vi "Update Plugin Types.vi"(8 "error in (no error)":errorcluster, 10 "plugin_types":T1[](array[typedef]), 11 "Plugin Types ref in":refnum<vi>) -> (0 "error out":errorcluster, 3 "Plugin Types ref out":refnum<vi>)   [LabVIEW 2021, in "CIF_UI.lvclass"]
uses:
  CIF_UI.lvclass
  CIF_UI.lvclass/CIF_UI.ctl
  CIFPluginManager/CIFPluginManager/gRPC/CIF_Manager_client/RPC Messages/cif_manager_PluginVersion.ctl
  CIFPluginManager/CIFPluginManager/gRPC/CIF_Manager_client/CIF_Manager_client.lvlib
  CIFPluginManager/CIFPluginManager/gRPC/CIF_Manager_client/RPC Messages/cif_manager_PluginType.ctl
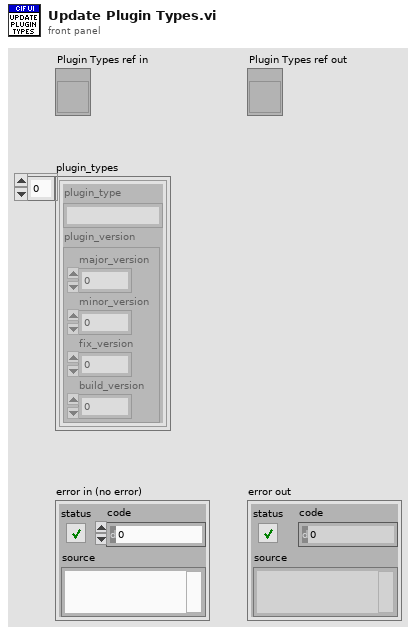
[diagram p1: front panel]
types:
  T1 = typedef "CIF_Manager_client.lvlib/cif_manager_PluginType.ctl" = cluster{"plugin_type":string, "plugin_version":T2}
  T2 = typedef "CIF_Manager_client.lvlib/cif_manager_PluginVersion.ctl" = cluster{"major_version":i32, "minor_version":i32, "fix_version":i32, "build_version":i32}
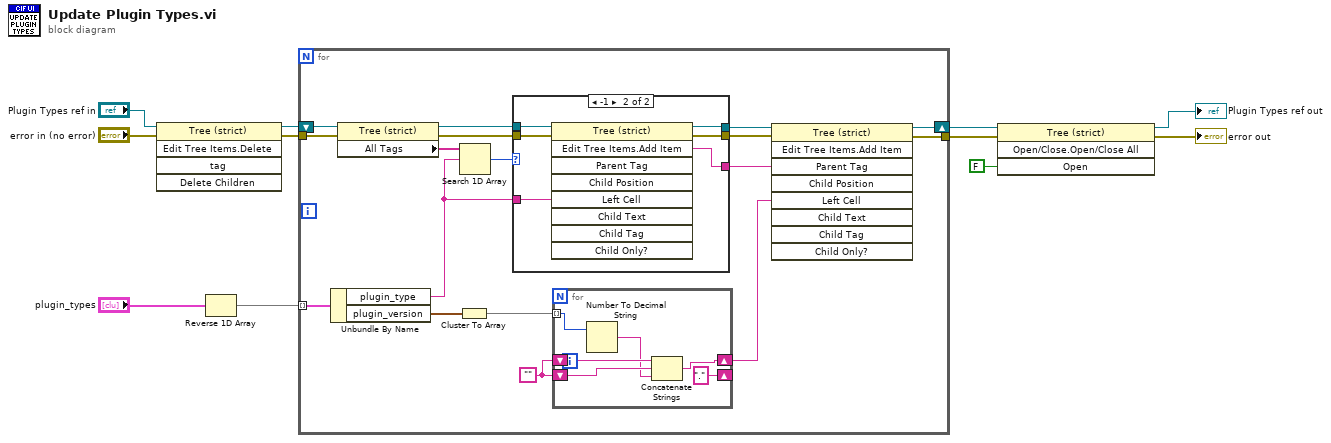
[diagram p0: block diagram]
diagram:
  n1 = invoke class="Tree (strict)" method="Edit Tree Items.Delete"(reference="Plugin Types ref in", error in="error in (no error)") -> (reference out=w10:refnum<vi>, error out=w11:errorcluster)  [unwired: 3 in, 3 out]
  n2 = Reverse 1D Array(array="plugin_types") -> (reversed array=w1:T1[])
  n3 = for {
    tunnel: w11 -> [w17]
    tunnel: [w27] -> w8
    tunnel: w1 -> [w25] mode=indexing
    shift-right: [w12] -> w9
    shift-left: w10 -> [w18]
    w22 = ""
    n4 = Unbundle By Name(w25) -> ("plugin_type"=w20:string, "plugin_version"=w24:T2)
    n5 = property class="Tree (strict)"(reference=w18, error in=w17) -> (reference out=w14:refnum<vi>, error out=w16:errorcluster, "All Tags"=w15:string[])
    n6 = Cluster To Array(cluster=w24) -> (array=w23:i32[])
    n7 = Search 1D Array(1D array=w15, element=w20) -> (index of element=w19:i32)  [unwired: 1 in]
    n8 = case shown="-1" w19 {
      tunnel: [w30 w34] -> w28
      tunnel: [w31 w33] -> w26
      tunnel: w16 -> [w31 w37]
      tunnel: w20 -> [w30 w35]
      tunnel: w14 -> [w29 w36]
      tunnel: [w29 w32] -> w13
      frame 0, Default {
      }
      frame -1 {
        n9 = invoke class="Tree (strict)" method="Edit Tree Items.Add Item"(reference=w36, error in=w37, "Left Cell"=w35) -> (reference out=w32:refnum<vi>, error out=w33:errorcluster, "Edit Tree Items:Add Item"=w34:string)  [unwired: 6 in, 6 out]
      }
    }
    n10 = for {
      tunnel: w23 -> [w41] mode=indexing
      shift-right: ["."] -> _
      shift-left: w22 -> [w42]
      shift-right: [w39] -> w21
      shift-left: w22 -> [w43]
      n11 = Number To Decimal String(number=w41) -> (decimal integer string=w40:string)  [unwired: 1 in]
      n12 = Concatenate Strings(w43, w42, w40) -> (w39:string)
    }
    n13 = invoke class="Tree (strict)" method="Edit Tree Items.Add Item"(reference=w13, error in=w26, "Parent Tag"=w28, "Left Cell"=w21) -> (reference out=w12:refnum<vi>, error out=w27:errorcluster)  [unwired: 5 in, 7 out]
  }
  n14 = invoke class="Tree (strict)" method="Open/Close.Open/Close All"(reference=w9, error in=w8, "Open"=FALSE ("Open?")) -> (reference out=→"Plugin Types ref out":refnum<vi>, error out=→"error out":errorcluster)  [unwired: 1 in, 2 out]
